vi "Table_UI.vi"(5 "Sort Type":enum16{"numerical", "hex", "string"}(ring), 7 "Sort by":u16(ring) items=["Packet_Number", "Timestamp", "Source", "Destination", "Protocol", "Length", "Data"], 8 "Table Control":refnum<vi>, 9 "Unsorted Data":string[][](array[string]), 10 "Filter String":string="Protocol == UDP AND Length > 0.7 OR Source == 192.168.1.1", 11 "Headers":string[](array[string])=["Timestamp", "ID", "Type", "Dir", "DLC", "Data"]) -> (3 "Table Control":string[][](table))   [LabVIEW 2025, in "Table_Filtering.lvlib"]
uses:
  Table_Filtering.lvlib
panel:
  in  "error in":errorcluster
  out "error out":errorcluster
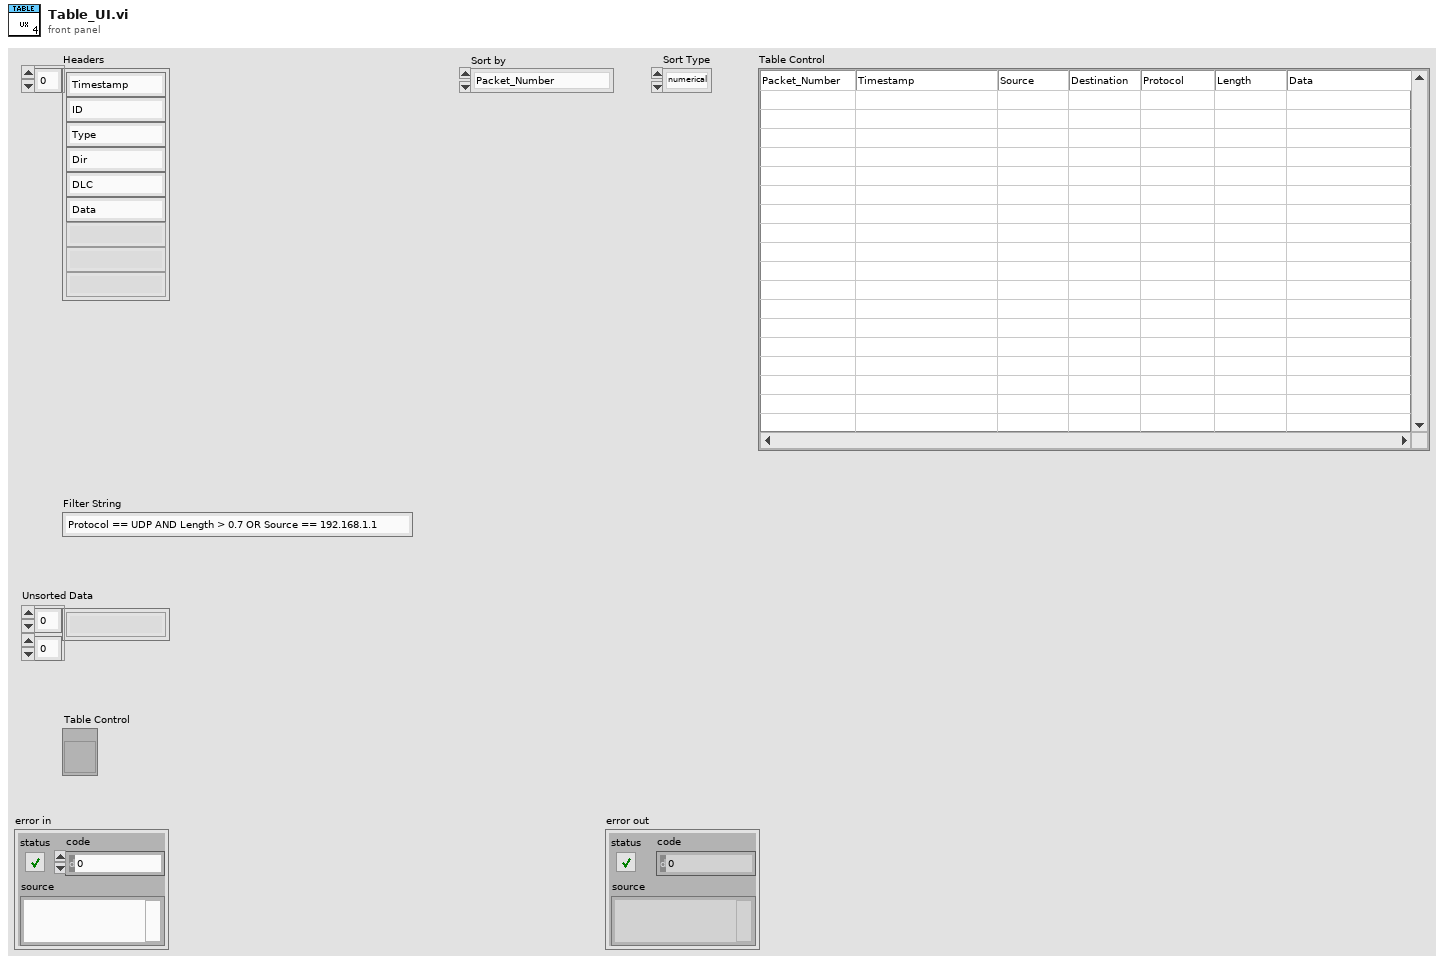
[diagram p1: front panel]
types:
  T1 = cluster{"FIELD":string, "OPERATOR":string, "VALUE":string}[]
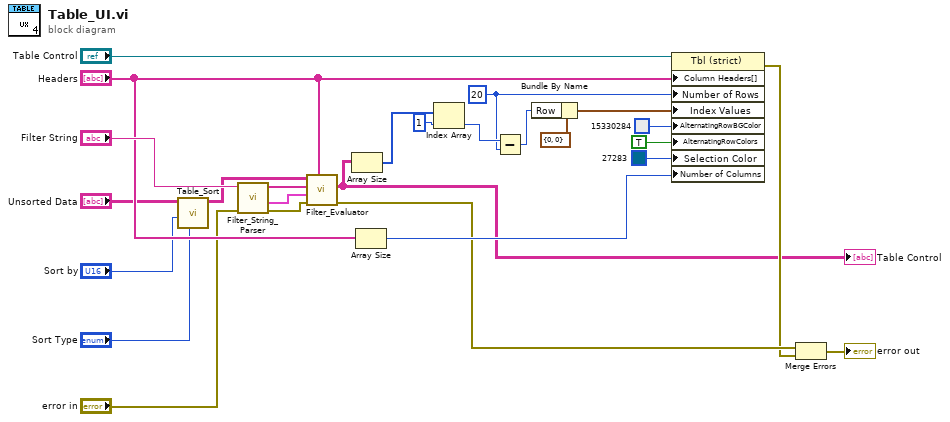
[diagram p0: block diagram]
diagram:
  w17 = 20 ("y")
  n1 = call "Table_Sort.vi"("Sort Type"="Sort Type", "Sort by"="Sort by", "Unsorted Data"="Unsorted Data") -> ("Sorted data"=w8:string[][])  [unwired: 8 in]
  n2 = call "Filter_String_Parser.vi"("error in"="error in", "Filter String"="Filter String") -> ("error constant"=w11:errorcluster, "Comparators"=w25:T1, "Boolean Connectors"=w24:string[])  [unwired: 7 in]
  n3 = call "Filter_Evaluator.vi"("Headers"="Headers", "Error"=w11, "Comparators"=w25, "Boolean Connectors"=w24, "Prefiltered Data"=w8) -> ("Error Out"=w5:errorcluster, "Filtered Array"=w1:string[][])  [unwired: 4 in, 1 out]
  "Table Control" <- w1
  n4 = Array Size(array=w1) -> (size(s)=w23:i32[])
  n5 = Array Size(array="Headers") -> (size(s)=w15:i32)
  n6 = Index Array(array=w23, index=1) -> (element=w22:i32)
  n7 = Subtract(x=w22, y=w17) -> (x-y=w21:i32)
  n8 = Bundle By Name(cluster=cluster{"Row":u32, "Column":u32} {"Row"=0, "Column"=0} ("Index Values"), "Row"=w21) -> (w18:cluster{"Row":u32, "Column":u32})
  n9 = property on="Property Node" class="Tbl (strict)"(reference="Table Control", "Column Headers[]"="Headers", "Number of Rows"=w17, "Index Values"=w18, "AlternatingRowBGColor"=u32 15330284 ("Alternate Row Background Color"), "AlternatingRowColors"=TRUE ("Alternating Row Colors"), "Selection Color"=u32 27283, "Number of Columns"=w15) -> (error out=w3:errorcluster)  [unwired: 1 in, 1 out]
  n10 = Merge Errors(w5, w3) -> (→"error out":errorcluster)
